vi "citTemplate.EnumDescriptorToArray.vi"(7 "enum type descriptor":string) -> (8 "array":string[](array[string]))   [LabVIEW 2019, in "Tools.lvlib"]
uses:
  Tools.lvlib
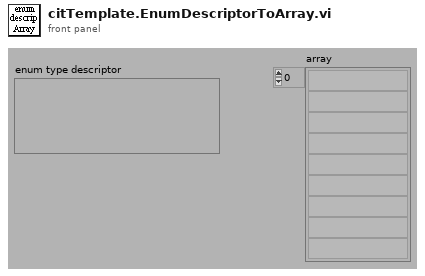
[diagram p1: front panel]
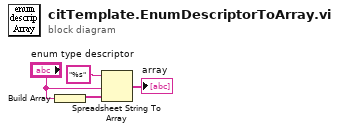
[diagram p0: block diagram]
diagram:
  n1 = Build Array("enum type descriptor") -> (w3:string[])
  n2 = Spreadsheet String To Array(format string="%s", spreadsheet string="enum type descriptor", array type (2D Dbl)=w3) -> (array=→"array":string[])  [unwired: 1 out]
